vi "ReadCode.vi"(8 "error in (no error)":errorcluster, 11 "object in":refnum<class "execute_request Message.lvclass">) -> (0 "error out":errorcluster, 2 "code":string, 3 "object out":refnum<class "execute_request Message.lvclass">)   [LabVIEW 2018, in "ClientMessaging.lvlib" / "execute_request Message.lvclass"]
uses:
  execute_request Message.lvclass
  execute_request Message.lvclass/execute_request Message.ctl
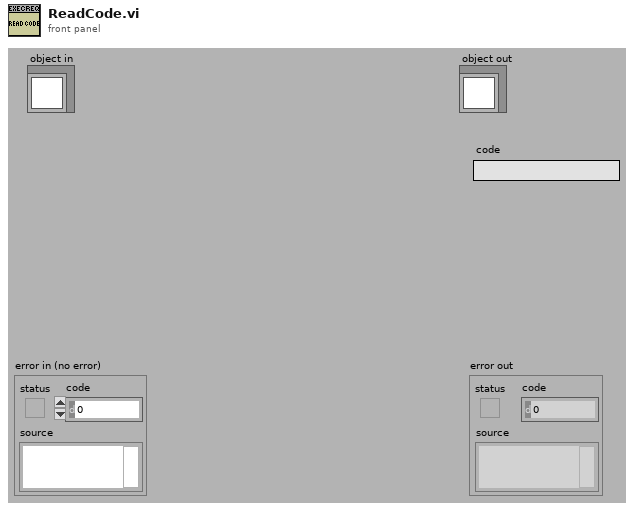
[diagram p1: front panel]
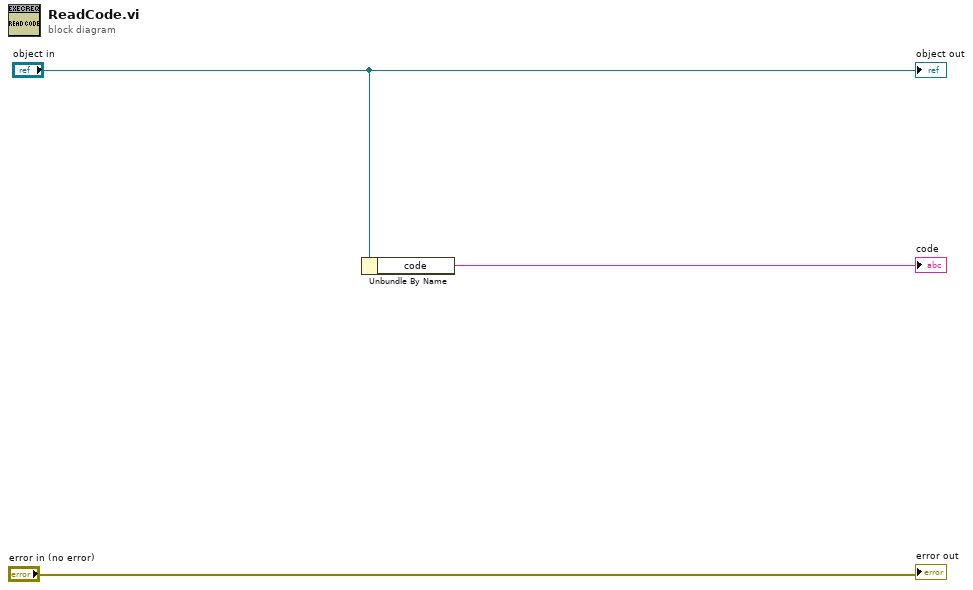
[diagram p0: block diagram]
diagram:
  n1 = Unbundle By Name("object in") -> ("code"=→"code":string)
  "error out" <- "error in (no error)"
  "object out" <- "object in"
